vi "updateCost&Price.vi"(0 "QBdata":string[][](array[string]), 1 "priceListData":string[][](array[string]), 2 "cost":dbl[][](array[numeric]), 3 "price":dbl[][](array[numeric]), 5 "error in (no error)":errorcluster, 10 "marketing&&service":bool) -> (16 "newQBdata":string[][](array[string]), 19 "error out":errorcluster)   [LabVIEW 2012]
uses:
  Controls/elaborationStatus.ctl
panel:
  out "String":string
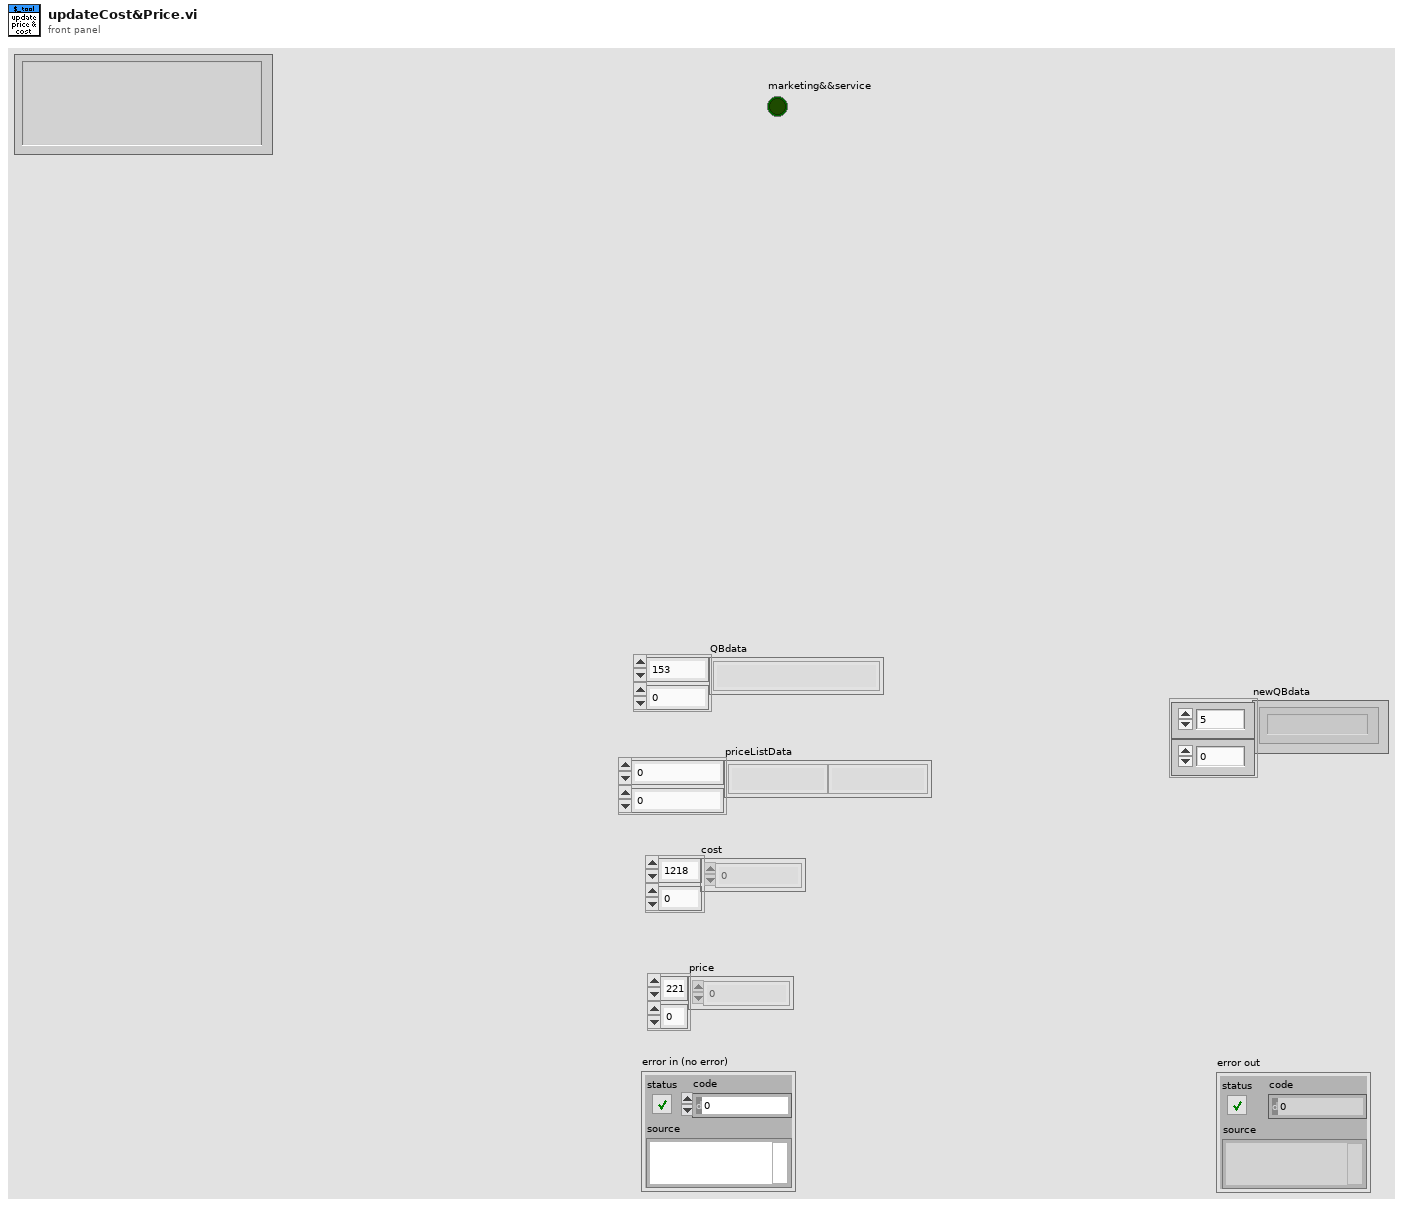
[diagram p1: front panel]
types:
  T1 = typedef "elaborationStatus.ctl" = enum16{"find", "notFound", "newItem", "update", "next item", "stop"}
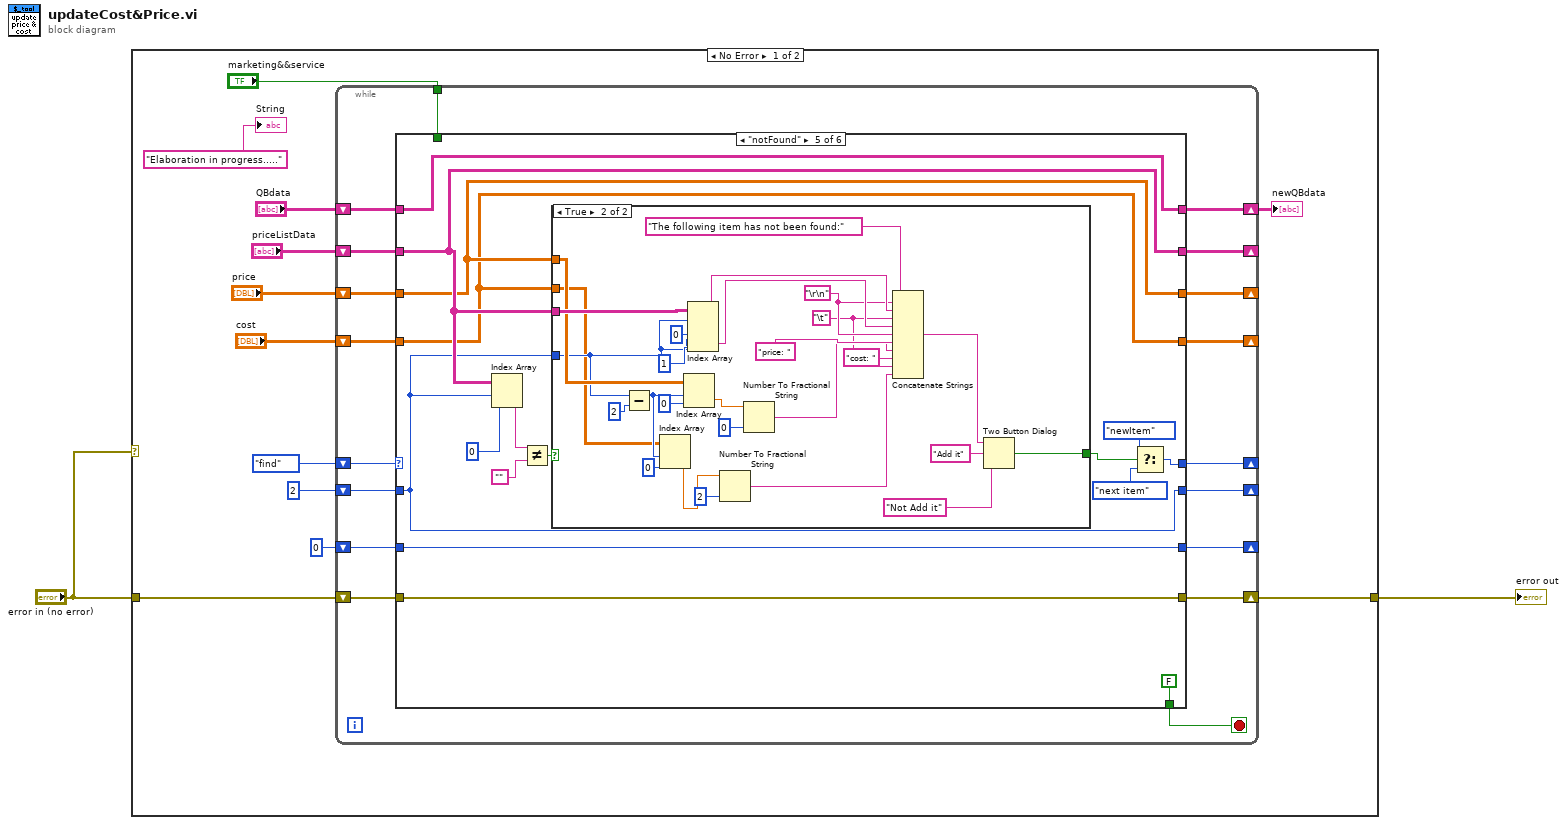
[diagram p0: block diagram]
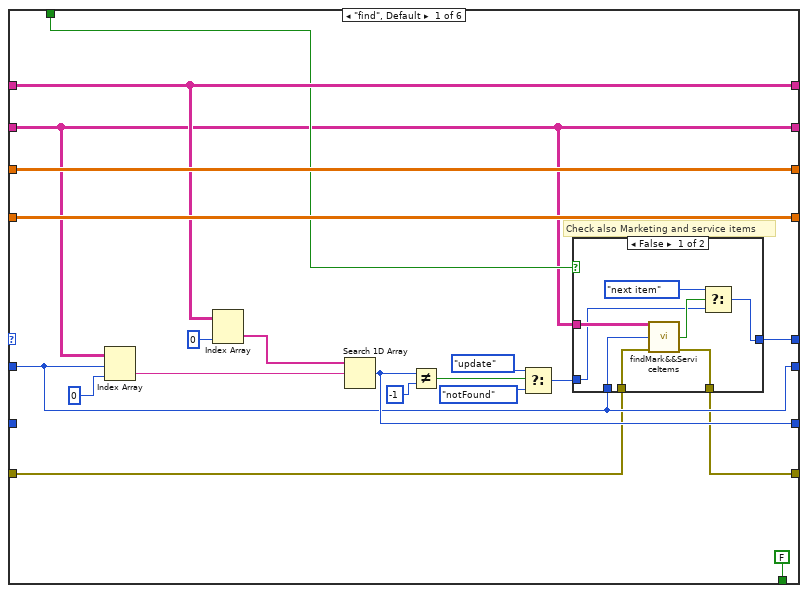
[diagram p2: hidden frame]
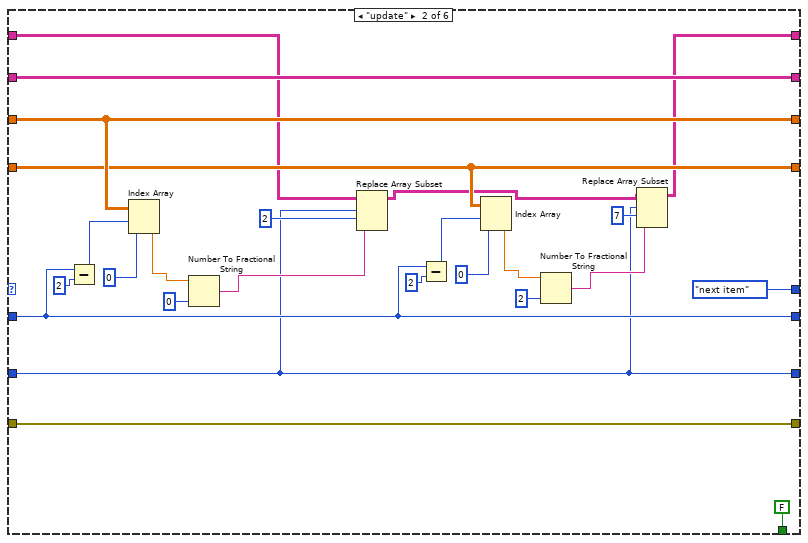
[diagram p4: hidden frame]
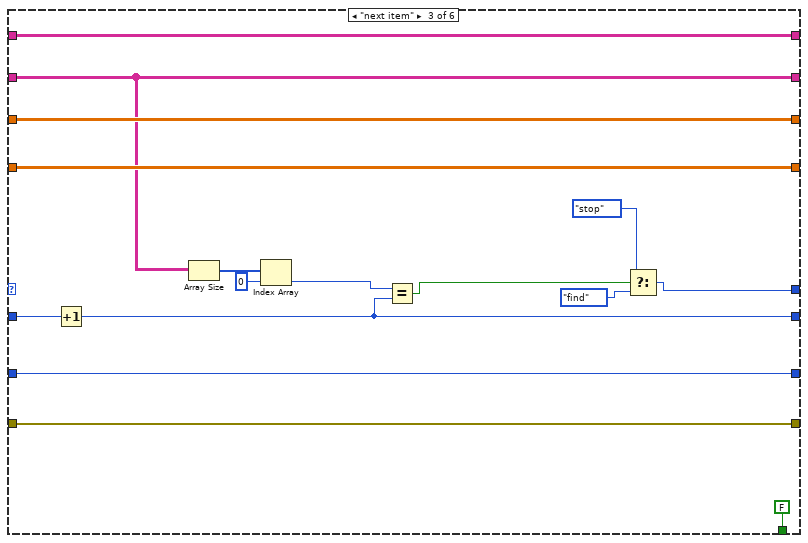
[diagram p5: hidden frame]
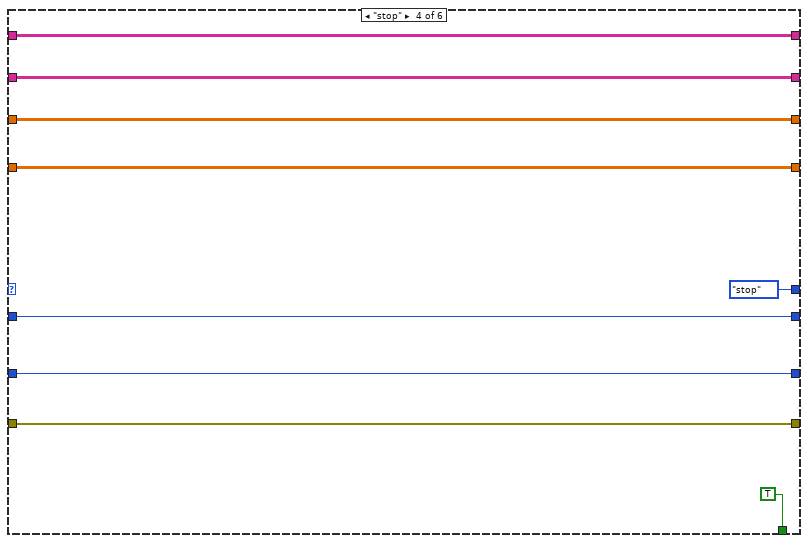
[diagram p6: hidden frame]
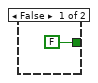
[diagram p7: hidden frame]
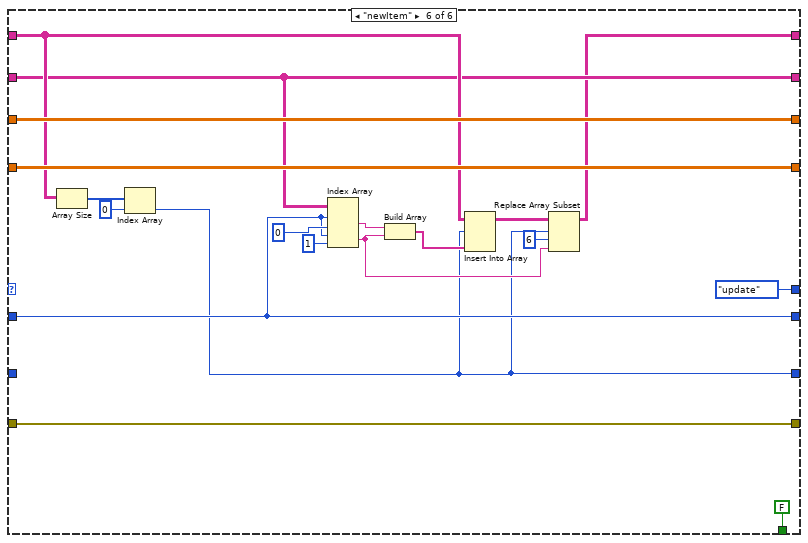
[diagram p8: hidden frame]
diagram:
  n1 = case shown="No Error" "error in (no error)" {
    tunnel: "error in (no error)" -> [w14 w176]
    tunnel: [w13 w176] -> w2
    frame No Error {
      n2 = while {
        shift-right: [w31] -> w13
        shift-left: w14 -> [w32]
        shift-right: [w28] -> w7
        shift-left: "QBdata" -> [w29]
        shift-right: [w26] -> _
        shift-left: "priceListData" -> [w27]
        shift-right: [w24] -> _
        shift-left: "price" -> [w25]
        shift-right: [w22] -> _
        shift-left: "cost" -> [w23]
        shift-right: [w20] -> _
        shift-left: elaborationStatus."find" ("elaboration_status") -> [w30]
        shift-right: [w17] -> _
        shift-left: 2 ("disabled index (col)") -> [w21]
        shift-right: [w19] -> _
        shift-left: 0 ("index of element") -> [w18]
        tunnel: "marketing&&service" -> [w15]
        stop <- w16 stop-if-true
        n3 = case shown="\"notFound\"" w30 {
          tunnel: w32 -> [w35 w87 w98 w106 w127 w173]
          tunnel: [w34 w87 w98 w106 w127 w173] -> w31
          tunnel: w29 -> [w48 w66 w103 w112 w122 w168]
          tunnel: [w48 w64 w103 w112 w122 w160] -> w28
          tunnel: w27 -> [w33 w86 w97 w111 w120 w166]
          tunnel: [w33 w86 w97 w111 w120 w166] -> w26
          tunnel: w25 -> [w52 w84 w102 w110 w118 w175]
          tunnel: [w52 w84 w102 w110 w118 w175] -> w24
          tunnel: w23 -> [w51 w67 w101 w109 w117 w174]
          tunnel: [w51 w67 w101 w109 w117 w174] -> w22
          tunnel: w21 -> [w36 w69 w100 w108 w119 w165]
          tunnel: [w37 elaborationStatus."next item" ("elaboration_status") w89 elaborationStatus."stop" ("elaboration_status") w114 elaborationStatus."update" ("elaboration_status")] -> w20
          tunnel: [w41 w68 w99 w107 w128 w157] -> w19
          tunnel: w18 -> [_ w68 w99 w107 w128 _]
          tunnel: [w36 w69 w93 w108 w119 w165] -> w17
          tunnel: [FALSE FALSE FALSE TRUE FALSE FALSE] -> w16
          tunnel: w15 -> [w38 _ _ _ _ _]
          frame "find", Default {
            # "Check also Marketing and service items"
            n4 = Index Array(array=w33, index (row)=w36, index (col)=0 ("disabled index (col)")) -> (element=w49:string)
            n5 = Index Array(array=w48, index (col)=0 ("disabled index (col)")) -> (element=w46:string[])  [unwired: 1 in]
            n6 = Search 1D Array(1D array=w46, element=w49) -> (index of element=w41:i32)  [unwired: 1 in]
            n7 = Not Equal?(x=w41, y=-1) -> (x != y?=w43:bool)
            n8 = Select(t=elaborationStatus."update" ("elaboration_status"), s=w43, f=elaborationStatus."notFound" ("elaboration_status")) -> (s? t:f=w39:T1)
            n9 = case shown="False" w38 {
              tunnel: w39 -> [w55 w62]
              tunnel: [w54 w62] -> w37
              tunnel: w36 -> [w58 _]
              tunnel: w35 -> [w60 w61]
              tunnel: [w59 w61] -> w34
              tunnel: w33 -> [w57 _]
              frame False {
                n10 = call "findMark&&ServiceItems.vi"("priceListData"=w57, "Numeric"=w58, "error in (no error)"=w60) -> ("found?"=w56:bool, "error IO"=w59:errorcluster)  [unwired: 11 in]
                n11 = Select(t=elaborationStatus."next item", s=w56, f=w55) -> (s? t:f=w54:T1)
              }
              frame True {
              }
            }
          }
          frame "update" {
            n12 = Subtract(x=w69, y=2) -> (x-y=w83:i32)
            n13 = Index Array(array=w84, index (row)=w83, index (col)=0 ("disabled index (col)")) -> (element=w79:dbl)
            n14 = Number To Fractional String(number=w79, precision (6)=i16 0) -> (F-format string=w78:string)  [unwired: 2 in]
            n15 = Replace Array Subset(array=w66, new element=w78, index (row)=w68, index (col)=2 ("disabled index (col)")) -> (w65:string[][])
            n16 = Subtract(x=w69, y=2) -> (x-y=w70:i32)
            n17 = Index Array(array=w67, index (row)=w70, index (col)=0 ("disabled index (col)")) -> (element=w74:dbl)
            n18 = Number To Fractional String(number=w74, precision (6)=i16 2) -> (F-format string=w75:string)  [unwired: 2 in]
            n19 = Replace Array Subset(array=w65, new element=w75, index (row)=w68, index (col)=7 ("disabled index (col)")) -> (w64:string[][])
          }
          frame "next item" {
            n20 = Increment(x=w100) -> (x+1=w93:i32)
            n21 = Array Size(array=w97) -> (size(s)=w96:i32[])
            n22 = Index Array(array=w96, index=0) -> (element=w94:i32)
            n23 = Equal?(x=w94, y=w93) -> (x = y?=w92:bool)
            n24 = Select(t=elaborationStatus."stop" ("elaboration_status"), s=w92, f=elaborationStatus."find" ("elaboration_status")) -> (s? t:f=w89:T1)
          }
          frame "stop" {
          }
          frame "notFound" {
            n25 = Index Array(array=w120, index (row)=w119, index (col)=0 ("disabled index (col)")) -> (element=w124:string)
            n26 = Not Equal?(x=w124, y="") -> (x != y?=w121:bool)
            n27 = case shown="True" w121 {
              tunnel: w120 -> [_ w152]
              tunnel: w119 -> [_ w139]
              tunnel: w118 -> [_ w140]
              tunnel: w117 -> [_ w132]
              tunnel: [FALSE ("T button?") w138] -> w116
              frame False {
              }
              frame True {
                w130 = "\t"
                w147 = "\r\n"
                n28 = Subtract(x=w139, y=2) -> (x-y=w133:i32)
                n29 = Index Array(array=w132, index (row)=w133, index (col)=0 ("disabled index (col)")) -> (element=w136:dbl)
                n30 = Index Array(array=w140, index (row)=w133, index (col)=0 ("disabled index (col)")) -> (element=w141:dbl)
                n31 = Index Array(array=w152, index (row) #1=w139, index (col) #1=0 ("disabled index (col)"), index (row) #2=w139, index (col) #2=1 ("disabled index (col)")) -> (element #1=w149:string, element #2=w148:string)
                n32 = Number To Fractional String(number=w136, precision (6)=i16 2) -> (F-format string=w131:string)  [unwired: 2 in]
                n33 = Number To Fractional String(number=w141, precision (6)=i16 0) -> (F-format string=w137:string)  [unwired: 2 in]
                n34 = Concatenate Strings("The following item has not been found:" ("string"), w147, w149, w130, w148, w147, "price: " ("string"), w137, w130, "cost: " ("string"), w131) -> (w155:string)
                n35 = Two Button Dialog(message=w155, 1:"Not Add it" ("F button name (\"Cancel\")"), 2:"Add it" ("T button name (\"OK\")")) -> (T button?=w138:bool)
              }
            }
            n36 = Select(t=elaborationStatus."newItem" ("elaboration_status"), s=w116, f=elaborationStatus."next item" ("elaboration_status")) -> (s? t:f=w114:T1)
          }
          frame "newItem" {
            n37 = Array Size(array=w168) -> (size(s)=w170:i32[])
            n38 = Index Array(array=w170, index=0) -> (element=w157:i32)
            n39 = Index Array(array=w166, index (row) #1=w165, index (col) #1=0 ("disabled index (col)"), index (row) #2=w165, index (col) #2=1 ("disabled index (col)")) -> (element #1=w163:string, element #2=w158:string)
            n40 = Build Array(w163, w158) -> (w162:string[])
            n41 = Insert Into Array(array=w168, index (row)=w157, new element=w162) -> (w161:string[][])  [unwired: 1 in]
            n42 = Replace Array Subset(array=w161, new element=w158, index (row)=w157, index (col)=6 ("disabled index (col)")) -> (w160:string[][])
          }
        }
      }
      "newQBdata" <- w7
      "String" <- "Elaboration in progress....." ("String")
    }
    frame Error {
    }
  }
  "error out" <- w2
